vi "NCS_AmpPh.vi"(8 "IQ":cdb[](array[numeric]), 9 "data":cdb[][](array[numeric]), 10 "Sampling Rate":i32=500, 11 "Coerced Rx IQ Rate":dbl) -> (0 "Phase DownSampled":dbl[](array[numeric]), 1 "Amp DownSampled":dbl[](array[numeric]), 2 "Unfiltered Phase":dbl[](array[numeric]), 3 "Unfiltered Amplitude":dbl[](array[numeric]))   [LabVIEW 2016]
uses:
  <vilib>/Analysis/3filter.llb/Butterworth Filter (DBL).vi
  <vilib>/Analysis/NI_AALBase.lvlib
  <vilib>/Analysis/NI_AALPro.lvlib
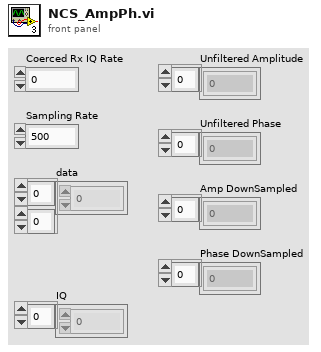
[diagram p1: front panel]
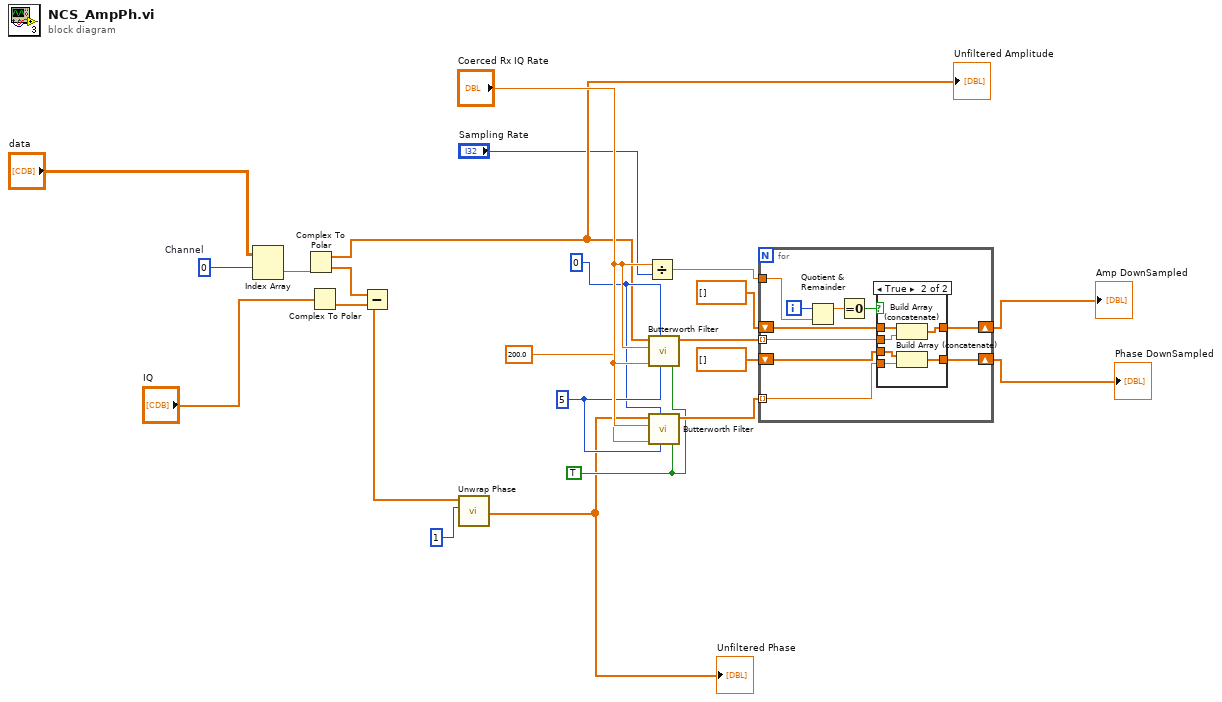
[diagram p0: block diagram]
diagram:
  w5 = 0  # Channel
  w16 = 5 ("order1")
  w21 = 200.0 ("Low-Pass Freq")
  w17 = TRUE
  w15 = 0
  n1 = Index Array(array="data", index (row)=w5) -> (element=w3:cdb[])  [unwired: 1 in]
  n2 = Complex To Polar(r * e^(i*theta)=w3) -> (r=w9:dbl[], theta=w14:dbl[])
  "Unfiltered Amplitude" <- w9
  n3 = Complex To Polar(r * e^(i*theta)="IQ") -> (theta=w12:dbl[])  [unwired: 1 out]
  n4 = Subtract(x=w14, y=w12) -> (x-y=w2:dbl[])
  n5 = call <vilib>:"Unwrap Phase.vi"("phase unit"=1 ("y"), "Phase"=w2) -> ("Unwrapped Phase"=w1:dbl[])  [unwired: 8 in, 1 out]
  "Unfiltered Phase" <- w1
  n6 = Divide(x="Coerced Rx IQ Rate", y="Sampling Rate") -> (x/y=w8:dbl)
  n7 = call-poly <vilib>:"Butterworth Filter.vi"("init/cont (init:F)"=w17, "order"=w16, "filter type"=w15, "low cutoff freq: fl"=w21, "sampling freq: fs"="Coerced Rx IQ Rate", "X"=w9) -> ("Filtered X"=w10:dbl[])  [unwired: 2 in, 1 out]
  n8 = call-poly <vilib>:"Butterworth Filter.vi"("init/cont (init:F)"=w17, "order"=w16, "filter type"=w15, "low cutoff freq: fl"=w21, "sampling freq: fs"="Coerced Rx IQ Rate", "X"=w1) -> ("Filtered X"=w19:dbl[])  [unwired: 2 in, 1 out]
  n9 = for {
    tunnel: w10 -> [w33] mode=indexing
    shift-right: [w31] -> w22
    shift-left: dbl[] [] -> [w32]
    tunnel: w8 -> [w27]
    shift-right: [w25] -> w20
    shift-left: dbl[] [] -> [w26]
    tunnel: w19 -> [w24] mode=indexing
    i -> [w30]
    n10 = Quotient & Remainder(x=w30, y=w27) -> (x-y*floor(x/y)=w28:dbl)  [unwired: 1 out]
    n11 = Equal To 0?(x=w28) -> (x = 0?=w29:bool)
    n12 = case shown="True" w29 {
      tunnel: w33 -> [_ w41]
      tunnel: w32 -> [w35 w40]
      tunnel: [w35 w39] -> w31
      tunnel: w26 -> [w34 w38]
      tunnel: [w34 w37] -> w25
      tunnel: w24 -> [_ w36]
      frame False {
      }
      frame True {
        n13 = Build Array (concatenate)(w40, w41) -> (w39:dbl[])
        n14 = Build Array (concatenate)(w38, w36) -> (w37:dbl[])
      }
    }
  }
  "Amp DownSampled" <- w22
  "Phase DownSampled" <- w20
